vi "Control To Private Data.vi"(9 "Ctl Refnum":refnum<vi>, 10 "User VI Ref":refnum<vi>) -> ()   [LabVIEW 2021]
uses:
  _Control To Private Data/_Control To Private Data.lvlib
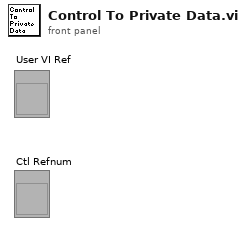
[diagram p1: front panel]
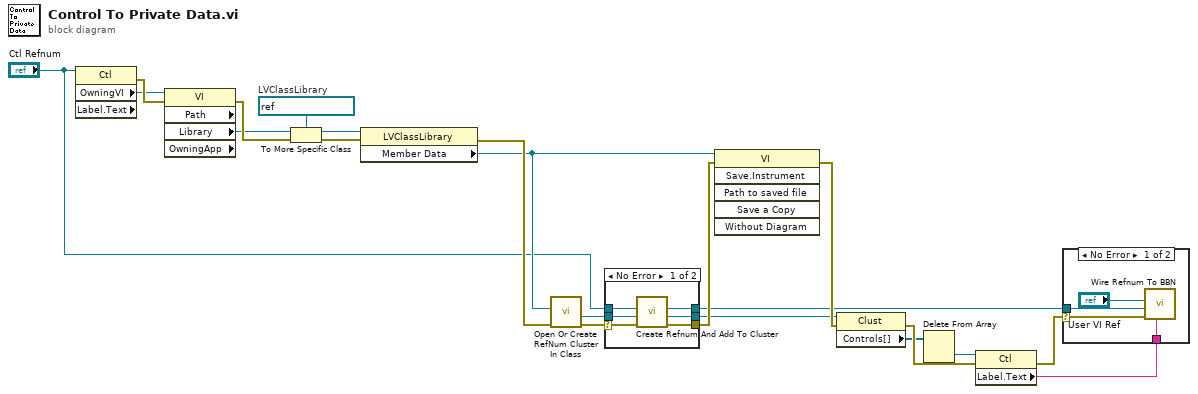
[diagram p0: block diagram]
diagram:
  w10 = refnum<vi> refnum  # LVClassLibrary
  n1 = property class="Ctl" props=["OwningVI", "Label", "Text"](reference="Ctl Refnum") -> (error out=w21:errorcluster, "OwningVI"=w12:refnum<vi>)  [unwired: 1 in, 2 out]
  n2 = property class="VI" props=["Path", "Library", "OwningApp"](reference=w12, error in=w21) -> (error out=w19:errorcluster, "Library"=w11:refnum<vi>)  [unwired: 3 out]
  n3 = To More Specific Class(target class=w10, reference=w11, error in=w19) -> (specific class reference=w9:refnum<vi>, error out=w20:errorcluster)
  n4 = property class="LVClassLibrary"(reference=w9, error in=w20) -> (error out=w16:errorcluster, "Member Data"=w2:refnum<vi>)  [unwired: 1 out]
  n5 = call "Open Or Create RefNum Cluster In Class.vi"("error in"=w16, "VI in"=w2) -> ("error out"=w15:errorcluster, "Cluster out"=w6:refnum<vi>)  [unwired: 8 in]
  n6 = case shown="No Error" w15 {
    selector: w15 -> [w27 w28]
    tunnel: [w26 w28] -> w14
    tunnel: w6 -> [w25 w29]
    tunnel: [w24 w29] -> w5
    tunnel: "Ctl Refnum" -> [w23 _]
    tunnel: [w22 _] -> w3
    frame No Error {
      n7 = call "Create Refnum And Add To Cluster.vi"("error in"=w27, "Owning Cluster in"=w25, "Ctl Refnum"=w23) -> ("error out"=w26:errorcluster, "Owning Cluster out"=w24:refnum<vi>, "Created RefNum"=w22:refnum<vi>)  [unwired: 6 in]
    }
    frame Error {
    }
  }
  n8 = invoke class="VI" method="Save.Instrument"(reference=w2, error in=w14) -> (error out=w18:errorcluster)  [unwired: 4 in, 5 out]
  n9 = property class="Clust"(reference=w5, error in=w18) -> (error out=w17:errorcluster, "Controls[]"=w8:refnum<vi>[])  [unwired: 1 out]
  n10 = Delete From Array "Delete From Array"(array=w8) -> (deleted portion=w7:refnum<vi>)  [unwired: 2 in, 1 out]
  n11 = property class="Ctl"(reference=w7, error in=w17) -> (error out=w13:errorcluster, "Label.Text"=w4:string)  [unwired: 1 out]
  n12 = case shown="No Error" w13 {
    selector: w13 -> [w33 _]
    tunnel: w4 -> [w32 _]
    tunnel: w3 -> [w31 _]
    frame No Error {
      n13 = call "Wire Refnum To BBN.vi"("Label.Text"=w32, "error in"=w33, "Created RefNum"=w31, "VI in"="User VI Ref") -> ()  [unwired: 8 in]
    }
    frame Error {
    }
  }
